vi "Bounds Intersect.vi"(10 "Bounds 2":T1, 11 "Bounds 1":T1) -> (3 "Intersect?":bool)   [LabVIEW 2019, in "2D.lvlib"]
doc: "Test if two bounding rectangles intersect. Returns true if they intersect, false otherwise."
uses:
  <vilib>/Utility/miscctls.llb/LVRectTypeDef.ctl
  2D.lvlib
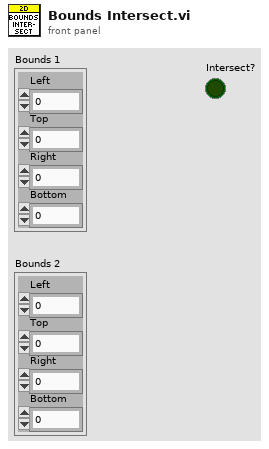
[diagram p1: front panel]
types:
  T1 = typedef "LVRectTypeDef.ctl" = cluster{"Left":i16, "Top":i16, "Right":i16, "Bottom":i16}
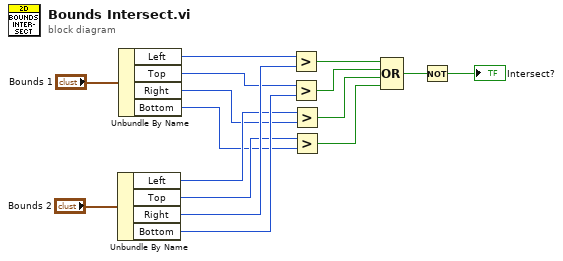
[diagram p0: block diagram]
diagram:
  n1 = Unbundle By Name("Bounds 2") -> ("Left"=w10:i16, "Top"=w8:i16, "Right"=w13:i16, "Bottom"=w11:i16)
  n2 = Unbundle By Name("Bounds 1") -> ("Left"=w14:i16, "Top"=w12:i16, "Right"=w9:i16, "Bottom"=w7:i16)
  n3 = Greater?(x=w14, y=w13) -> (0:w6:bool)
  n4 = Greater?(x=w12, y=w11) -> (0:w5:bool)
  n5 = Greater?(x=w10, y=w9) -> (0:w4:bool)
  n6 = Greater?(x=w8, y=w7) -> (0:w3:bool)
  n7 = Compound Arithmetic op=OR(w6, w5, w4, w3) -> (w2:bool)
  n8 = Not(x=w2) -> (.not. x?=→"Intersect?":bool)
